vi "Untitled 7.vi"   [LabVIEW 2018]
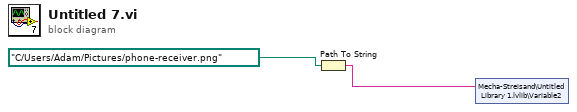
[diagram p0: block diagram]
diagram:
  n1 = Path To String(path=path "C:/Users/Adam/Pictures/phone-receiver.png") -> (string=w1:string)
  n2 = shared-variable "Mecha-Streisand\\Untitled Library 1.lvlib\\Variable2"(w1) -> ()  [unwired: 1 in, 1 out]
